vi "configureFilter.vi"(8 "error in (no error)":errorcluster, 11 "ElectrometerController in":refnum<class "ElectrometerController.lvclass">) -> (0 "error out":errorcluster, 1 "MedianFilter":bool, 2 "AVG Filter type":bool, 3 "ElectrometerController out":refnum<class "ElectrometerController.lvclass">, 4 "Filter":bool)   [LabVIEW 2016, in "ElectrometerController.lvclass"]
uses:
  ElectrometerController.lvclass
  ts_sallv_calibrationelectrometer/DataTypes/command_SetDigitalFilter.ctl
  Electrometer/AVG Filter type.ctl
  ElectrometerController.lvclass/ElectrometerController.ctl
  Electrometer/Electrometer.lvclass
  ElectrometerConfiguration/ElectrometerInternalConfiguration.lvclass
  Electrometer/State/ElectrometerState.lvclass
  ts_sallv_calibrationelectrometer/SALLV_calibrationElectrometer.lvlib
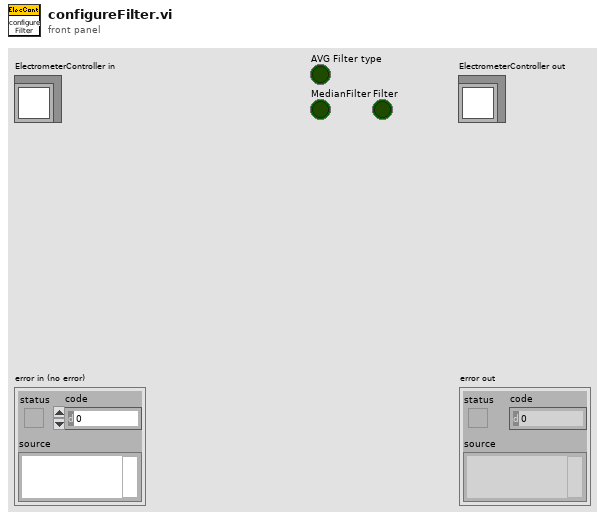
[diagram p1: front panel]
types:
  T1 = typedef "Electrometer.lvclass/AVG Filter type.ctl" = enum16{"None", "Scalar", "Advanced"}
  T2 = typedef "SALLV_calibrationElectrometer.lvlib/command_SetDigitalFilter.ctl" = cluster{"activateFilter":bool, "averageFilter":u16, "electId":i16, "medianFilter":bool}
  T3 = typedef "Electrometer.lvclass/MED Filter Type.ctl" = enum16{"Active", "None"}
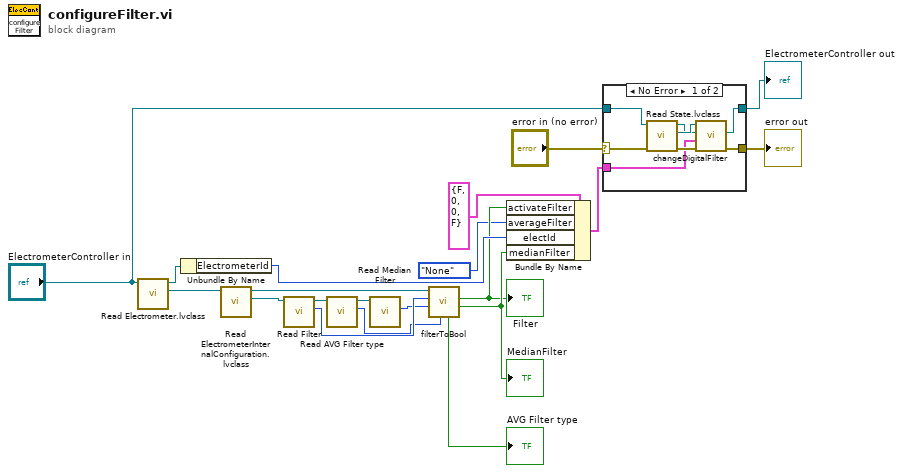
[diagram p0: block diagram]
diagram:
  n1 = call-dynamic "Read Electrometer.lvclass.vi"("ElectrometerController in"="ElectrometerController in") -> ("Electrometer.lvclass"=w18:refnum<class "Electrometer.lvclass">, "ElectrometerController out"=w6:refnum<class "ElectrometerController.lvclass">)  [unwired: 8 in, 1 out]
  n2 = Unbundle By Name(w6) -> ("ElectrometerId"=w5:enum16{"", "ID1", "ID2"})
  n3 = call-dynamic "Read ElectrometerInternalConfiguration.lvclass.vi"("Electrometer in"=w18) -> ("ElectrometerInternalConfiguration.lvclass"=w14:refnum<class "ElectrometerInternalConfiguration.lvclass">, "Electrometer out"=w13:refnum<class "Electrometer.lvclass">)  [unwired: 8 in, 1 out]
  n4 = call-dynamic "Read Filter.vi"("ElectrometerInternalConfiguration in"=w14) -> ("Filter"=w12:T3, "ElectrometerInternalConfiguration out"=w15:refnum<class "ElectrometerInternalConfiguration.lvclass">)  [unwired: 8 in, 1 out]
  n5 = call-dynamic "Read AVG Filter type.vi"("ElectrometerInternalConfiguration in"=w15) -> ("AVG Filter type"=w10:T1, "ElectrometerInternalConfiguration out"=w16:refnum<class "ElectrometerInternalConfiguration.lvclass">)  [unwired: 8 in, 1 out]
  n6 = call-dynamic "Read Median Filter.vi"("ElectrometerInternalConfiguration in"=w16) -> ("Filter"=w11:T3)  [unwired: 8 in, 2 out]
  n7 = call "filterToBool.vi"("AVG Filter type"=w10, "MedianFilter"=w11, "Filter"=w12, "Electrometer in"=w13) -> ("MedianFilter"=w4:bool, "Filter"=w3:bool, "AVG Filter type"=→"AVG Filter type":bool)  [unwired: 3 in, 2 out]
  "MedianFilter" <- w4
  "Filter" <- w3
  n8 = Bundle By Name(cluster=T2 {"activateFilter"=FALSE, "averageFilter"=0, "electId"=0, "medianFilter"=FALSE} ("command_SetDigitalFilter"), "activateFilter"=w3, "averageFilter"=AVG_Filter_type."None" ("AVG Filter type"), "electId"=w5, "medianFilter"=w4) -> (w1:T2)
  n9 = case shown="No Error" "error in (no error)" {
    selector: "error in (no error)" -> [w25 w30]
    tunnel: [w24 w30] -> w19
    tunnel: [w22 w29] -> w17
    tunnel: "ElectrometerController in" -> [w23 w29]
    tunnel: w1 -> [w21 _]
    frame No Error {
      n10 = call-dynamic "Read State.lvclass.vi"("error in (no error)"=w25, "ElectrometerController in"=w23) -> ("error out"=w26:errorcluster, "ElectrometerState"=w28:refnum<class "ElectrometerState.lvclass">, "ElectrometerController out"=w27:refnum<class "ElectrometerController.lvclass">)  [unwired: 7 in]
      n11 = call-dynamic "changeDigitalFilter.vi"("error in (no error)"=w26, "command_SetDigitalFilter"=w21, "ElectrometerController in"=w27, "State in"=w28) -> ("error out"=w24:errorcluster, "ElectrometerController out"=w22:refnum<class "ElectrometerController.lvclass">)  [unwired: 5 in, 1 out]
    }
    frame Error {
    }
  }
  "error out" <- w19
  "ElectrometerController out" <- w17
